vi "CryoServer Shutdown.vi"(8 "error in (no error)":errorcluster, 11 "CryoServer in":refnum<class "CryoServer.lvclass">) -> (0 "error out":errorcluster, 3 "CryoServer out":refnum<class "CryoServer.lvclass">)   [LabVIEW 2019]
uses:
  CryoServer.lvclass
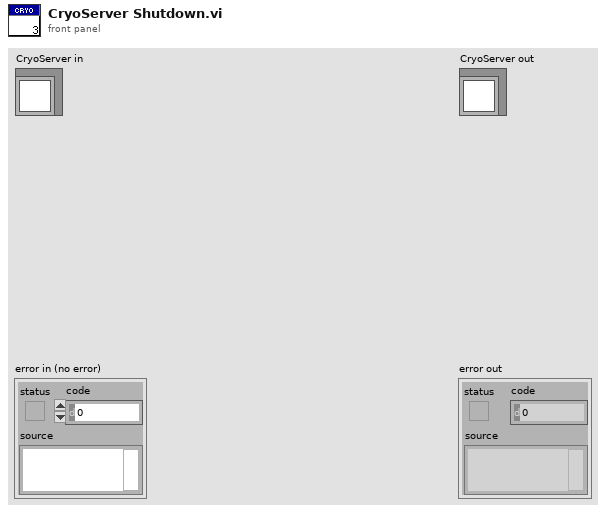
[diagram p1: front panel]
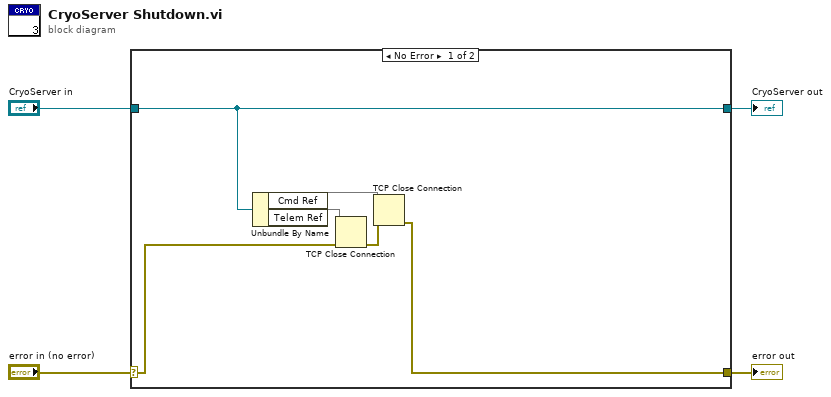
[diagram p0: block diagram]
diagram:
  n1 = case shown="No Error" "error in (no error)" {
    selector: "error in (no error)" -> [w6 w12]
    tunnel: [w5 w12] -> w3
    tunnel: [w10 w11] -> w1
    tunnel: "CryoServer in" -> [w10 w11]
    frame No Error {
      n2 = Unbundle By Name(w10) -> ("Cmd Ref"=w9, "Telem Ref"=w7)
      n3 = TCP Close Connection(connection ID=w7, error in (no error)=w6) -> (error out=w8:errorcluster)  [unwired: 1 in, 1 out]
      n4 = TCP Close Connection(connection ID=w9, error in (no error)=w8) -> (error out=w5:errorcluster)  [unwired: 1 in, 1 out]
    }
    frame Error {
    }
  }
  "error out" <- w3
  "CryoServer out" <- w1
